vi "manual_single_trigger.vi"   [LabVIEW 2011]
doc: "if this VI is executed, it triggers TRIG 1 via software once"
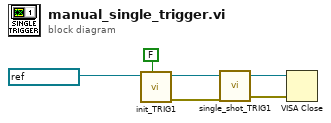
[diagram p0: block diagram]
diagram:
  n1 = call "init_TRIG1.vi"("reset"=FALSE ("reset TRIG"), "VISA resource name"=refnum<visa-resource-name> "TRIG1") -> ("error out"=w3:errorcluster, "VISA resource name out"=w4:refnum<visa-resource-name>)  [unwired: 8 in]
  n2 = call "single_shot_TRIG1.vi"("error in (no error)"=w3, "VISA resource name"=w4) -> ("error out"=w1:errorcluster, "VISA resource name 2"=w2:refnum<visa-resource-name>)  [unwired: 2 in]
  n3 = VISA Close(VISA resource name=w2, error in (no error)=w1) -> ()  [unwired: 1 out]
